vi "FPGA - Revert (ECAT).vi"(8 "error in (no error)":errorcluster, 11 "Node Ptr":u64 format="%.0x") -> (0 "error out":errorcluster)   [LabVIEW 2016, in "Scan Engine Custom Device.lvlib"]
uses:
  Scan Engine Custom Device.lvlib
panel:
  in  "Tag":string
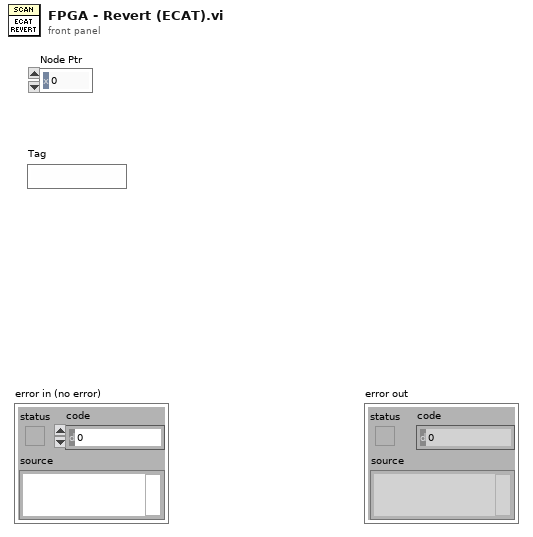
[diagram p1: front panel]
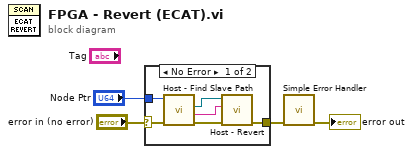
[diagram p0: block diagram]
diagram:
  n1 = case shown="No Error" "error in (no error)" {
    selector: "error in (no error)" -> [w7 w11]
    tunnel: "Node Ptr" -> [w5 _]
    tunnel: [w6 w11] -> w2
    frame No Error {
      n2 = call "Host - Find Slave Path.vi"("error in (no error)"=w7, "Item Ref in"=w5) -> ("error out"=w8:errorcluster, "Target IP Address"=w10:string, "Slave Ref"=w9:refnum<k21>)  [unwired: 6 in, 1 out]
      n3 = call "Host - Revert.vi"("error in"=w8, "Target IP Address in"=w10, "Slave Ref in"=w9) -> ("error out"=w6:errorcluster)  [unwired: 6 in, 2 out]
    }
    frame Error {
    }
  }
  n4 = call <vilib>:"Simple Error Handler.vi"("error in (no error)"=w2) -> ("error out"=→"error out":errorcluster)  [unwired: 4 in, 4 out]
